vi "TDC_Interface.vi"(0 "VISA resource name":refnum<visa-resource-name>="COM3", 1 "baud rate":u32=1000000, 2 "data bits":u16=8 min=5 max=8 step=1, 3 "parity":u16(ring) items=["None", "Odd", "Even", "Mark", "Space"], 4 "stop bits":u16(ring)=10 items=["1.0"=10, "1.5"=15, "2.0"=20], 7 "flow control":u16(ring) items=["None"=0, "XON/XOFF"=1, "RTS/CTS"=2, "DTR/DSR"=4]) -> ()   [LabVIEW 2013]
doc: "The Basic Serial Read and Write example performs a Serial Port Read, a Serial Port Write, or a combination of these actions. The user selects the actions (read or write) on the front panel. If both are selected, the VI will write the data first, read data, and then close the VISA session that is opened to the port. This VI will wait until the specified number of bytes is received at the port. Only the number of bytes specified will be read.\n\nINSTRUCTIONS:\n1) Select the serial resource and configuration parameters (baud rate, data bits, parity, stop bits, flow control).\n2) Select the operations to be performed. \n3) Connect the serial port to your device. If no device is available, perform a loopback test by doing one of the following. Short pins 2 and 3 on a RS-232 cable or short pin 4 to pin 8 and pin 5 to pin 9 on a RS-485/422 cable. \n4) Run the VI to see the data read. (The \"read string\" will match the \"string to write\" if a loopback test was performed.)\n\nNote: The parameters set for the serial port must match the parameters of the connected instrument or device. In this example, the bytes to read parameter specifies the number of bytes that the serial port reads. If there were more bytes at the port than the number specified in bytes to read, those bytes would not be read. Also, if you specify to read more bytes than the number of bytes actually read, you might receive a timeout error message.\n\nOn the block diagram, the Configure Serial Port VI sets the configuration parameters. The front panel displays the controls used to configure the basic parameters, such as baud rate, data bits, and parity. Constants configure the other parameters the user probably does not need set. After the VISA Configure Serial Port VI opens the VISA session and configures the port, the VI passes the VISA resource name to other VIs that perform operations on that VISA resource. The VISA Write function sends a command to the serial device and the VISA Read function returns data based on the command. The VISA Close function then closes the reference to the serial device. It is important to close the reference; otherwise communication through with that port through protocols other than VISA might not be possible."
uses:
  subvis/TDCdata.ctl
  <vilib>/Platform/TimedLoop/XDataNode/nitl_modes.ctl
  <vilib>/Platform/TimedLoop/XDataNode/timing_clust.ctl
  <vilib>/Platform/TimedLoop/XDataNode/wakeup.ctl
  <vilib>/Instr/_visa.llb/VISA Configure Serial Port (Instr).vi
  <vilib>/Utility/file.llb/Write To Spreadsheet File (string).vi
  <vilib>/Utility/file.llb/Write To Spreadsheet File (DBL).vi
  <vilib>/platform/TimedLoop/XDataNode/XDataNode.xnode
  <vilib>/Platform/TimedLoop/XDataNode/XDNodeRunTimeDep.lvlib
  <vilib>/Analysis/NI_AALPro.lvlib
  <vilib>/ptbypt/NI_PtbyPt.lvlib
panel:
  in  "Stop":bool
  in  "Plot last N results:":u32
  out "Startup test":bool
  out "Start tick count":u32
  out "Counts this iteration":i32
  out "Data Array":T1[](array[typedef])
  out "Num results":u16
  in  "Reset":bool
  in  "X Scale":enum16{"Raw ticks", "Calibrated time"}(ring)
  out "Temp (C)":sgl format="%#_5g"
  out "rest of the binary string":string
  out "return count":u32
  out "Calibration":cluster{dbl, "Temp (C)":sgl}(graph)
  in  "Calibrate every":dbl[unit]=5.0 caption="Time Target (s)"
  out "Resonator cal":sgl
  out "Calibration cycles":u16
  out "Tref":sgl[unit]
  out "Resonator, theor":sgl
  out "Clock factor":u8
  out "Cal":bool
  out "FIFO full":bool
  out "Arduino buffer full":bool
  in  "Avg. over":u32
  out "Count Rate":cluster{dbl[unit], dbl[unit], dbl[unit]}(knob)={0.0, 1480.394893080054, 1841.3125659545085} scale=0.0..5000.0 scale format="%#.5g"
  out "Counts":i32
  out "Time":dbl[unit] format="%#_4g"
  in  "Note for filename":string
  in  "Save data collected up to now":bool
  in  "Y Scale":enum16{"Log", "Linear"}(ring)
  out "Histogram of last N results:":cluster{"Axis":dbl[], "Histogram":i32[]}(graph)
  in  "X Max":dbl
  in  "X Min":dbl
  in  "# of bins:":dbl=20.0
  out "Results outside view:":cluster{"total":i32, "below":i32, "above":i32}
  out "Cycle Factor":dbl[unit] format="%#_5g"
  # "Set \"VISA resource name\" the Arduino's COM port. You can check this in Device Manager or in the Arduino IDE."
  # "Average"
  # "Instantaneous"
  # "Recent"
  # "A full buffer means some data was lost as the software cannot handle the count rate. This is not bad in itself, but continually full buffers may indicate a saturated photodetector or cause software stability problems. Decrease the light intensity."
  # "Data is saved in data/ under this VI's directory.\nThe filename contains the current date and time followed by the Note."
  # "Tick time is the calculated time resolution of the TDC (i.e., the width of each bin), based on configuration constants and the two calibration operations.\n\nTemperature is read from a digital sensor attached to the Arduino. This is an approximate reference only; it is not used in calibration."
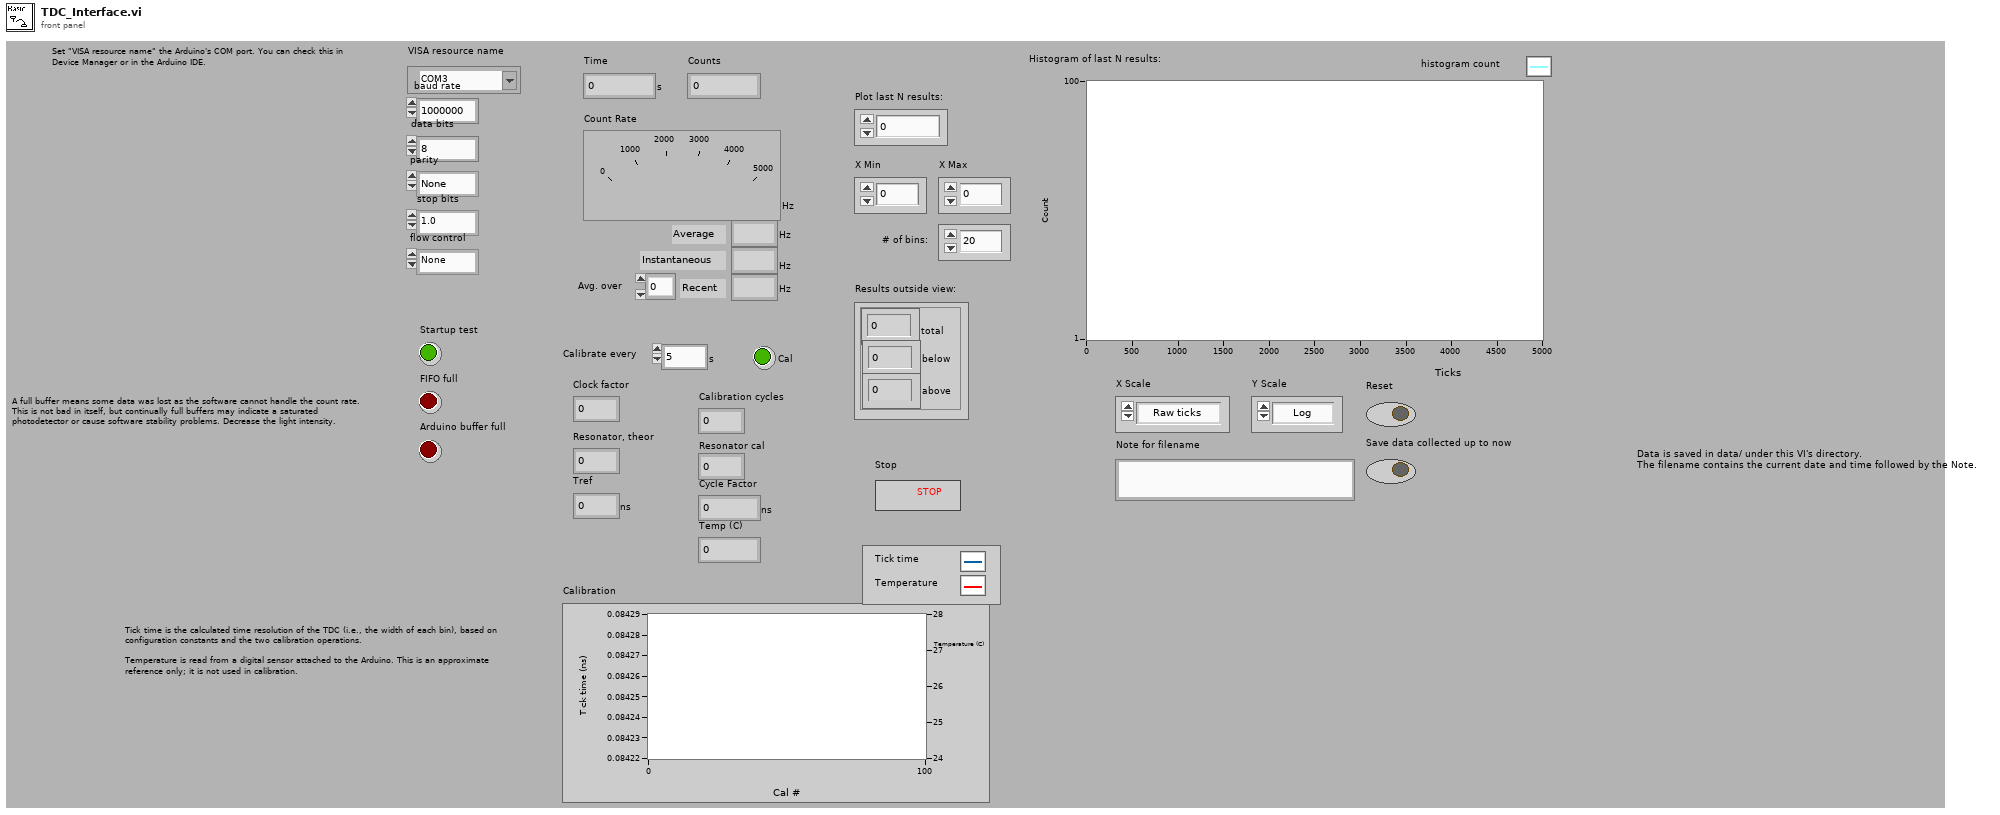
[diagram p1: front panel]
types:
  T1 = typedef "TDCdata.ctl" = cluster{"Ticks":i16, "Resonator cycles":sgl, "TDC cal cycles":u16, "Time (msec)":u32, "Temp (C)":sgl}
  T2 = typedef "XDNodeRunTimeDep.lvlib/nitl_modes.ctl" = enum32{"No Change", "Process missed periods, maintain original phase", "Discard missed periods, maintain original phase", "Process missed periods, ignore original phase", "Discard missed periods, ignore original phase"}
  T3 = typedef "XDNodeRunTimeDep.lvlib/timing_clust.ctl" = cluster{"Expected End [f-1]":u64, "Actual End [f-1]":u64, "Finished Late? [f-1]":bool, "Expected End [i-1]":u64, "Actual End [i-1]":u64, "Finished Late? [i-1]":bool, "Expected Start [i]":u64, "Actual Start [i]":u64, "Expected Start [f]":u64, "Actual Start [f]":u64, "Source Name":string, "Structure Name":string, "Period":i64, "Deadline":i64, "Offset":i64, "Start":i64, "Priority":i32, "Timeout":i32, "Mode":T2, "Wakeup Reason":T4, "Error":errorcluster, "Source Type":string, "Secondary Source Type":string, "Global End Time":u64, "Global Start Time":u64, "Frame Duration":u64, "Iteration Duration":u64, "Assigned CPU":i32, "I/O Scan Engine Mode":u32}
  T4 = typedef "XDNodeRunTimeDep.lvlib/wakeup.ctl" = enum32{"Normal", "Aborted", "Asynchronous wakeup", "Timing source error", "Timed loop error", "Timeout"}
  T5 = enum16{"big-endian, network order", "native, host order", "little-endian"}
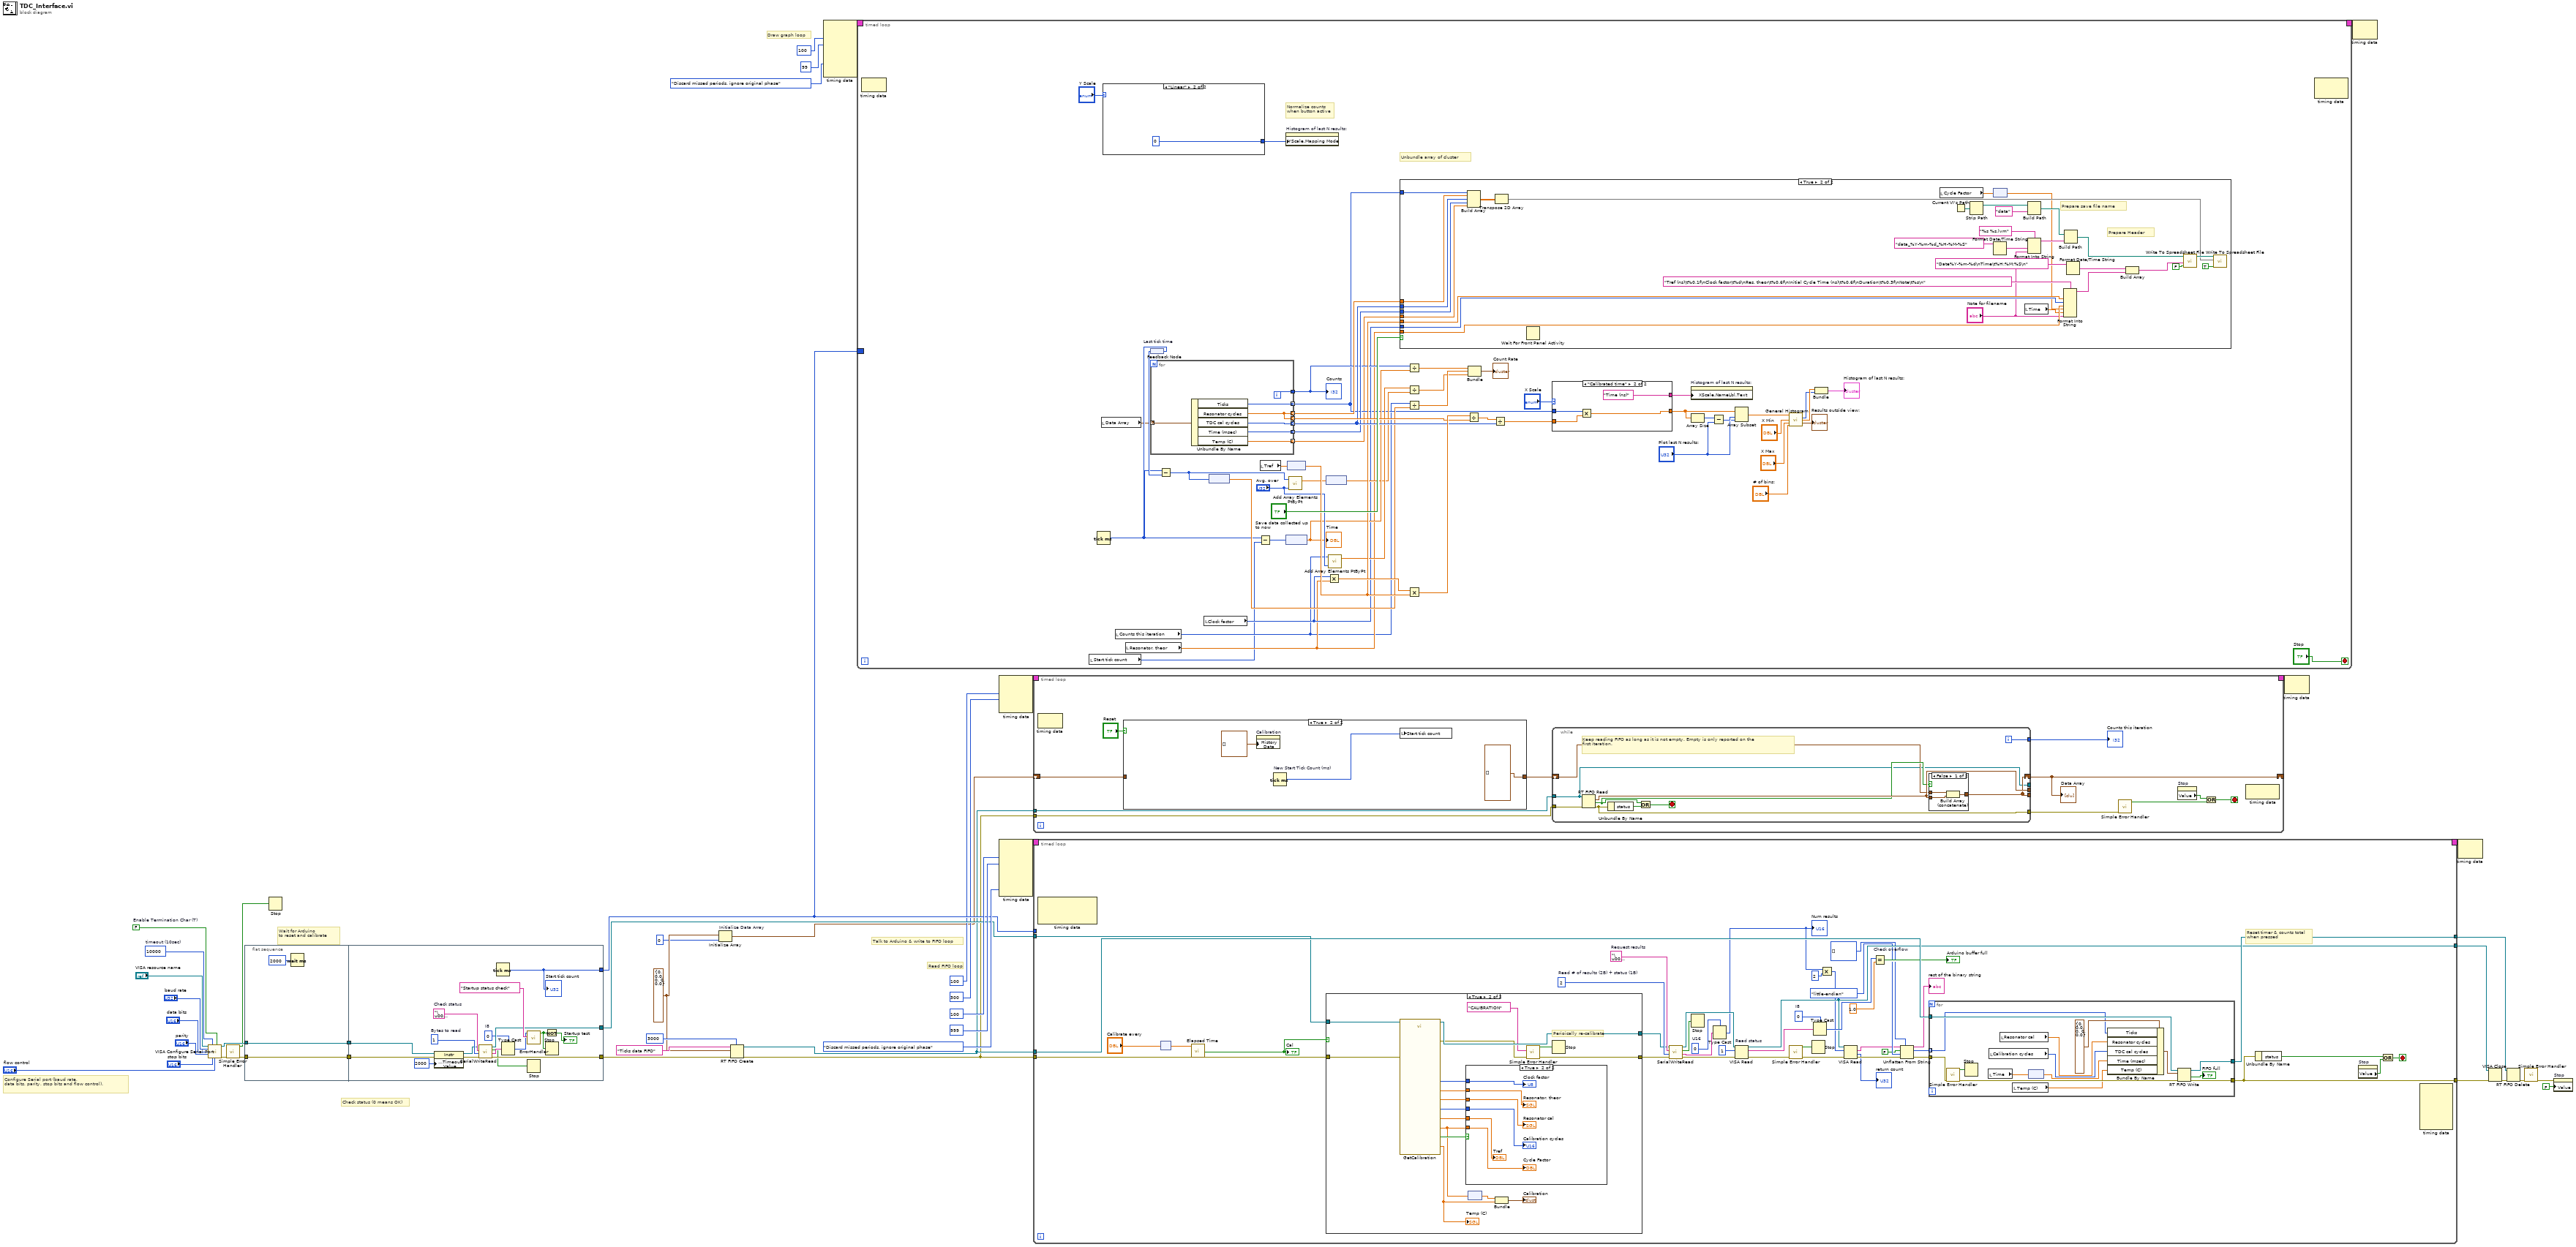
[diagram p0: block diagram]
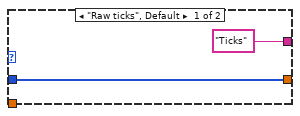
[diagram p4: hidden frame]
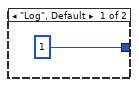
[diagram p6: hidden frame]
diagram:
  w14 = T1 {"Ticks"=0, "Resonator cycles"=0.0, "TDC cal cycles"=0, "Time (msec)"=0, "Temp (C)"=0.0} ("TDC data cluster")
  w41 = FALSE  # Enable Termination Char (T)
  w42 = u32 10000  # timeout (10sec)
  # "Read FIFO loop"
  # "Draw graph loop"
  # "Talk to Arduino & write to FIFO loop"
  # "Check status (0 means OK)"
  # "Wait for Arduino\nto reset and calibrate"
  # "Configure Serial port (baud rate,\ndata bits, parity, stop bits and flow control)."
  n1 = call-poly "VISA Configure Serial Port"("VISA resource name"="VISA resource name", "timeout (10sec)"=w42, "Enable Termination\nChar (T)"=w41, "baud rate (9600)"="baud rate", "data bits (8)"="data bits", "parity (0:none)"="parity", "stop bits (10: 1 bit)"="stop bits", "flow control (0:none)"="flow control") -> ("VISA resource name out"=w33:refnum<visa-resource-name>, "error out"=w27:errorcluster)  [unwired: 6 in]
  n2 = call <vilib>:"Simple Error Handler.vi"("error in (no error)"=w27) -> ("error?"=w25:bool, "error out"=w26:errorcluster)  [unwired: 4 in, 3 out]
  n3 = flat-sequence {
    tunnel: w33 -> [w48]
    tunnel: [w48] -> w32
    tunnel: [w46] -> w31
    tunnel: w26 -> [w46]
    tunnel: [w64] -> w19
    tunnel: [w63] -> w11
    tunnel: w32 -> [w55]
    tunnel: w31 -> [w53]
    tunnel: [w51] -> w10
    frame #0 {
      n4 = Wait (ms)(milliseconds to wait=u32 2000) -> ()  [unwired: 1 out]
    }
    frame #1 {
      w59 = u32 1  # Bytes to read
      w60 = "\u0000"  # Check status
      w62 = i8 0  # I8
      n5 = property class="Instr"(reference=w55, error in=w53, "General Settings:Timeout Value"=u32 2000) -> (reference out=w54:refnum<visa-resource-name>, error out=w52:errorcluster)
      n6 = call "SerialWriteRead.vi"("error in (no error)"=w52, "Bytes to read"=w59, "The byte to send before reading"=w60, "VISA Refnum in"=w54) -> ("error out"=w64:errorcluster, "Hex Out"=w61:string, "Error? Out"=w58:bool, "VISA Refnum out"=w63:refnum<visa-resource-name>)  [unwired: 4 in]
      n7 = Tick Count (ms)() -> (millisecond timer value=w51:u32)
      "Start tick count" <- w51
      n8 = Type Cast(type=w62, x=w61) -> (*(type *) &x=w57:i8)
      n9 = call "ErrorHandler.vi"("[error source]"="Startup status check" ("error source (\" \")"), "[error code]"=w57) -> ("error?"=w50:bool)  [unwired: 8 in, 1 out]
      n10 = Stop(stop? (T)=w58) -> ()
      n11 = Not(x=w50) -> (.not. x?=→"Startup test":bool)
      n12 = Stop(stop? (T)=w50) -> ()
    }
  }
  n13 = Stop(stop? (T)=w25) -> ()
  n14 = Initialize Array "Initialize Data Array"(w14, 0 ("size (10)")) -> (w3:T1[])
  n15 = RT FIFO Create(0:"Ticks data FIFO" ("name (unnamed)"), 1:w14, 3:w19, 4:u32 3000 ("size (10)")) -> (8:w5:refnum<k33>, 11:w4:errorcluster)  [unwired: 4 in, 1 out]
  n16 = node-c288(i64 100 ("Period"), 99 ("Priority"), nitl_modes."Discard missed periods, ignore original phase" ("Mode")) -> (w30:T3)  [unwired: 4 in]
  n17 = timed-loop {
    timing: w30 -> [_]
    timing-out: [_] -> w29
    border: w10 -> [_]
    stop <- "Stop" stop-if-true
    # "Unbundle array of cluster"
    # "Normalize counts\nwhen button active"
    n18 = node-c288() -> ()  [unwired: 1 in, 1 out]
    n19 = local read "Start tick count"() -> (w72:u32)
    n20 = Tick Count (ms)() -> (millisecond timer value=w81:u32)
    n21 = local read "Data Array"() -> (w73:T1[])
    n22 = case shown="\"Linear\"" "Y Scale" {
      tunnel: [1 0] -> w110
      frame "Log", Default {
      }
      frame "Linear" {
      }
    }
    n23 = local read "Counts this iteration"() -> (w74:i32)
    n24 = local read "Resonator, theor"() -> (w83:sgl)
    n25 = feedback-in #1(w81) -> ()
    n26 = feedback #1 "Last tick time"() -> (w82:u32)
    n27 = for {
      tunnel: w73 -> [w128] mode=indexing
      tunnel: [w126] -> w102 mode=indexing
      tunnel: [w127] -> w78 mode=indexing
      tunnel: [w126] -> w106 mode=indexing
      tunnel: [w125] -> w104 mode=indexing
      tunnel: [w124] -> w99 mode=indexing
      tunnel: [w123] -> w98
      tunnel: [w122] -> w75 mode=indexing
      i -> [w123]
      n28 = Unbundle By Name(w128) -> ("Ticks"=w127:i16, "Resonator cycles"=w126:sgl, "TDC cal cycles"=w125:u16, "Time (msec)"=w124:u32, "Temp (C)"=w122:sgl)
    }
    "Counts" <- w98
    n29 = Subtract(x=w81, y=w82) -> (x-y=w93:u32)
    n30 = local read "Clock factor"() -> (w85:u8)
    n31 = node(w93) -> (w90:dbl[unit])
    n32 = Subtract(x=w81, y=w72) -> (x-y=w97:u32)
    n33 = local read "Tref"() -> (w84:sgl[unit])
    n34 = property on="Histogram of last N results:" class="XYGraph (strict)"("YScale.Mapping Mode"=w110) -> ()  [unwired: 2 in, 2 out]
    n35 = node(w97) -> (w94:dbl[unit])
    "Time" <- w94
    n36 = node(w84) -> (w101:sgl)
    n37 = call <vilib>:"Add Array Elements PtByPt.vi"("sample length"="Avg. over", "input data point"=w93) -> ("sum"=w92:dbl)  [unwired: 2 in, 1 out]
    n38 = node(w92) -> (w91:dbl[unit])
    n39 = Multiply(x=w85, y=w83) -> (x*y=w105:sgl)
    n40 = call <vilib>:"Add Array Elements PtByPt.vi"("sample length"="Avg. over", "input data point"=w74) -> ("sum"=w95:dbl)  [unwired: 2 in, 1 out]
    n41 = case shown="True" "Save data collected up to now" {
      tunnel: w78 -> [_ w156]
      tunnel: w104 -> [_ w147]
      tunnel: w102 -> [_ w148]
      tunnel: w101 -> [_ w143]
      tunnel: w85 -> [_ w142]
      tunnel: w83 -> [_ w141]
      tunnel: w99 -> [_ w132]
      tunnel: w75 -> [_ w129]
      frame False {
      }
      frame True {
        # "Prepare Header"
        # "Prepare save file name"
        n42 = Build Array(w156, w148, w147, w132, w129) -> (w145:sgl[][])
        n43 = Transpose 2D Array(2D array=w145) -> (transposed array=w144:sgl[][])
        n44 = Wait For Front Panel Activity() -> ()  [unwired: 3 in, 1 out]
        n45 = local read "Cycle Factor"() -> (w131:dbl[unit])
        n46 = Current VI's Path() -> (path=w159:path)
        n47 = Strip Path(path=w159) -> (stripped path=w158:path)  [unwired: 1 out]
        n48 = node(w131) -> (w130:dbl)
        n49 = Format Date/Time String(time format string (%c)="data_%Y-%m-%d_%H-%M-%S") -> (date/time string=w133:string)  [unwired: 2 in]
        n50 = local read "Time"() -> (w138:dbl[unit])
        n51 = Build Path(base path=w158, name or relative path="data") -> (appended path=w151:path)
        n52 = Format Into String(format string="%s %s.lvm", w133, "Note for filename") -> (resulting string=w134:string)  [unwired: 2 in, 1 out]
        n53 = Format Into String(format string="Tref (ns)\t%0.1f\nClock factor\t%d\nRes. theor\t%0.6f\nInitial Cycle Time (ns)\t%0.6f\nDuration\t%0.3f\nNote\t%s\n" ("initial string"), w143, w142, w141, w130, w138, "Note for filename") -> (resulting string=w140:string)  [unwired: 2 in, 1 out]
        n54 = Build Path(base path=w151, name or relative path=w134) -> (appended path=w146:path)
        n55 = Format Date/Time String(time format string (%c)="Date%Y-%m-%d\nTime\t%H:%M:%S\n") -> (date/time string=w150:string)  [unwired: 2 in]
        n56 = Build Array(w150, w140) -> (w149:string[])
        n57 = call-poly <vilib>:"Write To Spreadsheet File.vi"("append to file? (new file:F)"=FALSE, "1D data"=w149, "file path (dialog if empty)"=w146) -> ("new file path (Not A Path if cancelled)"=w152:path)  [unwired: 5 in]
        n58 = call-poly <vilib>:"Write To Spreadsheet File.vi"("append to file? (new file:F)"=TRUE, "2D data"=w144, "file path (dialog if empty)"=w152) -> ()  [unwired: 5 in, 1 out]
      }
    }
    n59 = Divide(x=w98, y=w94) -> (x/y=w88:dbl[unit])
    n60 = Divide(x=w95, y=w91) -> (x/y=w86:dbl[unit])
    n61 = Divide(x=w74, y=w90) -> (x/y=w87:dbl[unit])
    n62 = Multiply(x=w105, y=w101) -> (x*y=w107:sgl)
    n63 = Divide(x=w107, y=w106) -> (x/y=w103:sgl[])
    n64 = Bundle(w88, w87, w86) -> (→"Count Rate":cluster{dbl[unit], dbl[unit], dbl[unit]})  [unwired: 1 in]
    n65 = Divide(x=w103, y=w104) -> (x/y=w79:sgl[])
    n66 = case shown="\"Calibrated time\"" "X Scale" {
      tunnel: w79 -> [_ w121]
      tunnel: w78 -> [w117 w120]
      tunnel: [w117 w119] -> w69
      tunnel: ["Ticks" ("X Scale.Name Label.Text") "Time (ns)" ("X Scale.Name Label.Text")] -> w77
      frame "Raw ticks", Default {
      }
      frame "Calibrated time" {
        n67 = Multiply(x=w120, y=w121) -> (x*y=w119:sgl[])
      }
    }
    n68 = property on="Histogram of last N results:" class="XYGraph (strict)"("XScale.NameLbl.Text"=w77) -> ()  [unwired: 2 in, 2 out]
    n69 = Array Size(array=w69) -> (size(s)=w71:i32)
    n70 = Subtract(x=w71, y="Plot last N results:") -> (x-y=w70:u32)
    n71 = Array Subset(array=w69, index=w70, length="Plot last N results:") -> (w68:sgl[])
    n72 = call <vilib>:"General Histogram.vi"("X"=w68, "max"="X Min", "min"="X Max", "# bins"="# of bins:") -> ("Histogram"=w76:i32[], "Axis"=w112:dbl[], "# outside"=→"Results outside view:":cluster{"total":i32, "below":i32, "above":i32})  [unwired: 7 in, 2 out]
    n73 = Bundle("Axis"=w112, "Histogram"=w76) -> (→"Histogram of last N results:":cluster{"Axis":dbl[], "Histogram":i32[]})  [unwired: 1 in]
    n74 = node-c288() -> ()  [unwired: 2 in, 1 out]
  }
  n75 = node-c288(i64 100 ("Period"), 300 ("Priority")) -> (w9:T3)  [unwired: 2 in]
  n76 = node-c288(i64 100 ("Period"), 999 ("Priority"), nitl_modes."Discard missed periods, ignore original phase" ("Mode")) -> (w36:T3)  [unwired: 4 in]
  n77 = timed-loop {
    timing: w9 -> [_]
    timing-out: [_] -> w8
    tunnel: w5 -> [w174]
    tunnel: w4 -> [w173]
    shift-right: [w171] -> _
    shift-left: w3 -> [w169]
    stop <- w164 stop-if-true
    n78 = node-c288() -> ()  [unwired: 1 in, 1 out]
    n79 = case shown="True" "Reset" {
      tunnel: [w175 T1[] []] -> w168
      tunnel: w169 -> [w175 _]
      frame False {
      }
      frame True {
        n80 = property on="Calibration" class="WFChart (strict)"("History Data"=cluster{dbl, sgl}[] []) -> ()  [unwired: 2 in, 2 out]
        n81 = Tick Count (ms) "New Start Tick Count (ms)"() -> (millisecond timer value=w176:u32)
        n82 = local write "Start tick count"(w176) -> ()
      }
    }
    n83 = while {
      tunnel: [w180] -> _
      tunnel: w173 -> [w188]
      tunnel: [w187] -> _
      shift-right: [w181] -> w171
      shift-left: w168 -> [w183]
      tunnel: [w182] -> w170
      tunnel: [w181] -> _
      tunnel: w174 -> [w180]
      tunnel: [w179] -> w172
      i -> [w182]
      stop <- w186 stop-if-true
      # "Keep reading FIFO as long as it is not empty. Empty is only reported on the \nfirst iteration."
      n84 = RT FIFO Read(0:w180, 3:w188) -> (9:w187:T1, 10:w184:bool, 11:w179:errorcluster)  [unwired: 2 in, 2 out]
      n85 = Unbundle By Name(w179) -> ("status"=w185:bool)
      n86 = Or(x=w184, y=w185) -> (x .or. y?=w186:bool)
      n87 = case shown="False" w184 {
        tunnel: w187 -> [w190 _]
        tunnel: w183 -> [w191 w192]
        tunnel: [w189 w192] -> w181
        frame False {
          n88 = Build Array (concatenate)(w191, w190) -> (w189:T1[])
        }
        frame True {
        }
      }
    }
    "Data Array" <- w171
    "Counts this iteration" <- w170
    n89 = call <vilib>:"Simple Error Handler.vi"("error in (no error)"=w172) -> ("error?"=w165:bool)  [unwired: 4 in, 4 out]
    n90 = property on="Stop" class="Bool (strict)"() -> ("Value"=w166:bool)  [unwired: 2 in, 2 out]
    n91 = Or(x=w166, y=w165) -> (x .or. y?=w164:bool)
    n92 = node-c288() -> ()  [unwired: 1 in, 1 out]
  }
  n93 = timed-loop {
    tunnel: w11 -> [w214]
    tunnel: w4 -> [w217]
    tunnel: [w220] -> w37
    timing: w36 -> [_]
    timing-out: [_] -> w35
    tunnel: [w210] -> w34
    tunnel: w10 -> [_]
    tunnel: w5 -> [w221]
    tunnel: [w219] -> w15
    stop <- w223 stop-if-true
    w236 = i8 0  # I8
    w231 = u32 2  # Read # of results (2B) + status (1B)
    w237 = u16 0  # U16
    w233 = "\u0002"  # Request results
    # "Reset timer & counts total\nwhen pressed"
    n94 = node-c288() -> ()  [unwired: 1 in, 3 out]
    n95 = node("Calibrate every") -> (w211:dbl)
    n96 = call "Elapsed Time"("Time Target (s)"=w211, "error in (no error)"=w217) -> ("Time has Elapsed"=w216:bool, "error out"=w215:errorcluster)  [unwired: 10 in, 6 out]
    "Cal" <- w216
    n97 = case shown="True" w216 {
      tunnel: [w239 w241] -> w196
      tunnel: w215 -> [w239 w256]
      tunnel: w214 -> [w238 w255]
      tunnel: [w238 w254] -> w213
      frame False {
      }
      frame True {
        # "Perioically re-calibrate"
        n98 = call "GetCalibration.vi"("VISA Refnum in"=w255, "error in (no error)"=w256) -> ("Temp (C)"=w240:sgl, "OK result"=w251:bool, "Tref"=w252:sgl[unit], "Cycle time"=w250:dbl[unit], "VISA Refnum out"=w254:refnum<visa-resource-name>, "Clock factor"=w253:u8, "Res. Theor. cycles"=w248:sgl, "Res. cycles"=w249:sgl, "TDC cycles"=w245:u16, "error out"=w244:errorcluster)  [unwired: 8 in]
        "Temp (C)" <- w240
        n99 = case shown="True" w251 {
          tunnel: w250 -> [_ w262]
          tunnel: w253 -> [_ w261]
          tunnel: w252 -> [_ w260]
          tunnel: w248 -> [_ w259]
          tunnel: w245 -> [_ w258]
          tunnel: w249 -> [_ w257]
          frame False {
          }
          frame True {
            "Cycle Factor" <- w262
            "Clock factor" <- w261
            "Resonator, theor" <- w259
            "Tref" <- w260
            "Calibration cycles" <- w258
            "Resonator cal" <- w257
          }
        }
        n100 = node(w250) -> (w247:dbl)
        n101 = Bundle(w247, "Temp (C)"=w240) -> (→"Calibration":cluster{dbl, "Temp (C)":sgl})  [unwired: 1 in]
        n102 = call <vilib>:"Simple Error Handler.vi"("error source (\" \")"="CALIBRATION" ("error source (\" \")"), "error in (no error)"=w244) -> ("error?"=w242:bool, "error out"=w241:errorcluster)  [unwired: 3 in, 3 out]
        n103 = Stop(stop? (T)=w242) -> ()
      }
    }
    n104 = call "SerialWriteRead.vi"("error in (no error)"=w196, "Bytes to read"=w231, "The byte to send before reading"=w233, "VISA Refnum in"=w213) -> ("error out"=w227:errorcluster, "Hex Out"=w230:string, "Error? Out"=w232:bool, "VISA Refnum out"=w226:refnum<visa-resource-name>)  [unwired: 4 in]
    n105 = Stop(stop? (T)=w232) -> ()
    n106 = Type Cast(type=w237, x=w230) -> (*(type *) &x=w200:u16)
    "Num results" <- w200
    n107 = VISA Read "Read status"(VISA resource name=w226, byte count=u32 1, error in (no error)=w227) -> (VISA resource name out=w210:refnum<visa-resource-name>, read buffer=w228:string, error out=w225:errorcluster)  [unwired: 1 out]
    n108 = call <vilib>:"Simple Error Handler.vi"("error in (no error)"=w225) -> ("error?"=w224:bool, "error out"=w209:errorcluster)  [unwired: 4 in, 3 out]
    n109 = Stop(stop? (T)=w224) -> ()
    n110 = Type Cast(type=w236, x=w228) -> (*(type *) &x=w234:i8)
    n111 = Multiply(x=w200, y=u32 2) -> (x*y=w199:u32)
    n112 = VISA Read(VISA resource name=w210, byte count=w199, error in (no error)=w209) -> (read buffer=w204:string, return count=→"return count":u32, error out=w207:errorcluster)  [unwired: 1 out]
    n113 = Equal? "Check overflow"(x=w234, y=1.0) -> (x = y?=→"Arduino buffer full":bool)
    n114 = Unflatten From String(type=u16[] [], binary string=w204, data includes array or string size? (T)=FALSE, byte order (0:big-endian, network order)=T5."little-endian", error in (no error)=w207) -> (rest of the binary string=→"rest of the binary string":string, value=w202:u16[], error out=w206:errorcluster)
    n115 = for {
      tunnel: [w273] -> w220
      tunnel: w221 -> [w275]
      tunnel: [w271] -> w219
      tunnel: w206 -> [w265]
      tunnel: w202 -> [w264] mode=indexing
      n116 = call <vilib>:"Simple Error Handler.vi"("error in (no error)"=w265) -> ("error?"=w277:bool, "error out"=w274:errorcluster)  [unwired: 4 in, 3 out]
      n117 = Stop(stop? (T)=w277) -> ()
      n118 = local read "Time"() -> (w267:dbl[unit])
      n119 = local read "Calibration cycles"() -> (w268:u16)
      n120 = local read "Resonator cal"() -> (w269:sgl)
      n121 = local read "Temp (C)"() -> (w263:sgl)
      n122 = node(w267) -> (w266:dbl)
      n123 = Bundle By Name(cluster=T1 {"Ticks"=0, "Resonator cycles"=0.0, "TDC cal cycles"=0, "Time (msec)"=0, "Temp (C)"=0.0} ("TDC data cluster 2"), "Ticks"=w264, "Resonator cycles"=w269, "TDC cal cycles"=w268, "Time (msec)"=w266, "Temp (C)"=w263) -> (w272:T1)
      n124 = RT FIFO Write(0:w275, 1:w272, 3:w274) -> (8:w271:refnum<k33>, 10:→"FIFO full":bool, 11:w273:errorcluster)  [unwired: 2 in, 1 out]
    }
    n125 = Unbundle By Name(w220) -> ("status"=w222:bool)
    n126 = property on="Stop" class="Bool (strict)"() -> ("Value"=w195:bool)  [unwired: 2 in, 2 out]
    n127 = Or(x=w222, y=w195) -> (x .or. y?=w223:bool)
    n128 = node-c288() -> ()  [unwired: 6 in, 1 out]
  }
  n129 = node-c288(w8) -> ()  [unwired: 1 out]
  n130 = node-c288(w29) -> ()  [unwired: 1 out]
  n131 = node-c288(w35) -> ()  [unwired: 1 out]
  n132 = VISA Close(VISA resource name=w34, error in (no error)=w37) -> (error out=w17:errorcluster)
  n133 = RT FIFO Delete(0:w15, 3:w17) -> (11:w16:errorcluster)  [unwired: 1 in]
  n134 = call <vilib>:"Simple Error Handler.vi"("error in (no error)"=w16) -> ("error out"=w1:errorcluster)  [unwired: 4 in, 4 out]
  n135 = property on="Stop" class="Bool (strict)"(error in=w1, "Value"=FALSE ("Stop")) -> ()  [unwired: 1 in, 2 out]
